vi "WT500 Integration Conditional Stop.vi"(8 "error in (no error)":errorcluster, 10 "Reset?":bool=TRUE, 11 "VISA Refnum in":refnum<visa-resource-name>) -> (0 "error out":errorcluster, 3 "VISA Refnum out":refnum<visa-resource-name>)   [LabVIEW 2012]
doc: "This VI query the Yokogawa WT500 to find out if it is integrating. If it is, it will stop and reset the ingration"
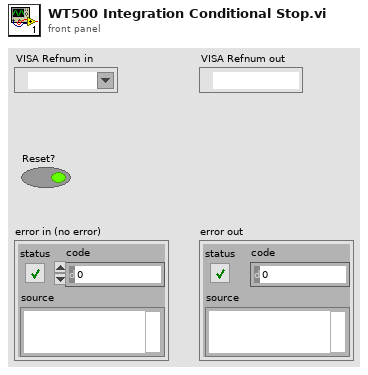
[diagram p1: front panel]
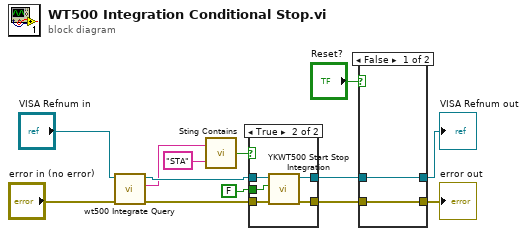
[diagram p0: block diagram]
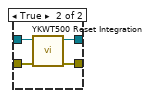
[diagram p2: hidden frame]
diagram:
  n1 = call "wt500 Integrate Query.vi"("error in (no error)"="error in (no error)", "VISA resource name"="VISA Refnum in") -> ("error out"=w12:errorcluster, "read buffer"=w8:string, "VISA resource name out"=w11:refnum<visa-resource-name>)  [unwired: 7 in]
  n2 = call "Sting Contains.vi"("Expression to evaluate"="STA", "Input String"=w8) -> ("Boolean"=w10:bool)
  n3 = case shown="True" w10 {
    tunnel: w11 -> [w15 w20]
    tunnel: w12 -> [w14 w19]
    tunnel: [w15 w17] -> w4
    tunnel: [w14 w16] -> w3
    tunnel: FALSE ("Start/Stop (False: Stop)") -> [_ w18]
    frame False {
    }
    frame True {
      n4 = call <instrlib>:"YKWT500 Start Stop Integration.vi"("error in (no error)"=w19, "Start/Stop (False: Stop)"=w18, "VISA resource name"=w20) -> ("error out"=w16:errorcluster, "VISA resource name out"=w17:refnum<visa-resource-name>)  [unwired: 7 in]
    }
  }
  n5 = case shown="False" "Reset?" {
    tunnel: w4 -> [w22 w26]
    tunnel: w3 -> [w21 w25]
    tunnel: [w22 w24] -> w1
    tunnel: [w21 w23] -> w2
    frame False {
    }
    frame True {
      n6 = call <instrlib>:"YKWT500 Reset Integration.vi"("error in (no error)"=w25, "VISA resource name"=w26) -> ("error out"=w23:errorcluster, "VISA resource name out"=w24:refnum<visa-resource-name>)  [unwired: 8 in]
    }
  }
  "error out" <- w2
  "VISA Refnum out" <- w1
